vi "ChooseDefensivePivot.vi"(1 "Defensive Driving Trigger":bool, 5 "Joystick Y":dbl, 6 "Joystick X":dbl) -> (0 "Pivot Module":i32)   [LabVIEW 2019]
doc: "***under development***"
uses:
  9a94878a-4914-4fba-839a-7657b048eec0.vi
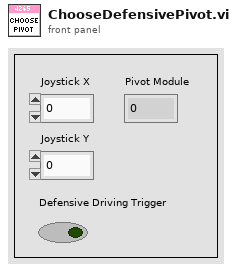
[diagram p1: front panel]
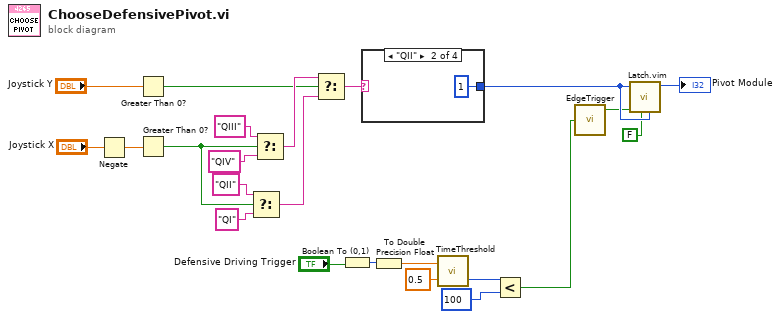
[diagram p0: block diagram]
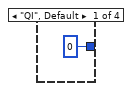
[diagram p2: hidden frame]
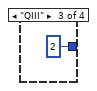
[diagram p3: hidden frame]
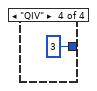
[diagram p4: hidden frame]
diagram:
  n1 = Negate(x="Joystick X") -> (-x=w13:dbl)
  n2 = Greater Than 0?(x="Joystick Y") -> (x > 0?=w16:bool)
  n3 = Greater Than 0?(x=w13) -> (x > 0?=w22:bool)
  n4 = Select(t="QII", s=w22, f="QI") -> (s? t:f=w23:string)
  n5 = Select(t="QIII", s=w22, f="QIV") -> (s? t:f=w18:string)
  n6 = Select(t=w18, s=w16, f=w23) -> (s? t:f=w1:string)
  n7 = Boolean To (0,1)(Boolean="Defensive Driving Trigger") -> (0, 1=w6:i16)
  n8 = case shown="\"QII\"" w1 {
    tunnel: [0 1 2 3] -> w11
    frame "QI", Default {
    }
    frame "QII" {
    }
    frame "QIII" {
    }
    frame "QIV" {
    }
  }
  n9 = To Double Precision Float(number=w6) -> (double precision float=w5:dbl)
  n10 = call "TimeThreshold.vi"("Threshold"=0.5, "Current Value"=w5) -> ("Time Below Threshold (ms)"=w4:u32)  [unwired: 1 out]
  n11 = Less?(x=w4, y=u32 100) -> (x < y?=w2:bool)
  n12 = call "EdgeTrigger.vi"("Input Signal"=w2) -> ("Rising Edge Trigger"=w10:bool)  [unwired: 2 out]
  n13 = call "Latch.vim"("Default Value"=w11, "Reset"=FALSE, "Latch Signal"=w10, "Latch Value"=w11) -> ("Latched"=→"Pivot Module":i32)  [unwired: 7 in]
